vi "AWG Write Multiple PreciseRamps From File.vi"(6 "SourceFolder Path":string, 8 "error in (no error)":errorcluster, 9 "AmpGain":i32=1, 10 "Channel Configurations":T2(array[cluster])=[{"PinNames"=["UP"], "WaveFormFile Name"=""}, {"PinNames"=["DOWN"], "WaveFormFile Name"=""}], 11 "Semiconductor Module Context":T1) -> (0 "error out":errorcluster)   [LabVIEW 2013]
uses:
  <vilib>/NI_TestStand_SemiconductorModule/NI_TestStand_Semiconductor_Module.lvlibp/PinMap/General/SemiconductorModuleContext.ctl
  <instrlib>/niFgen/niFgen.llb/niFgen Write Named Waveform (I16).vi
  <vilib>/NI_TestStand_SemiconductorModule/NI_TestStand_Semiconductor_Module.lvlibp
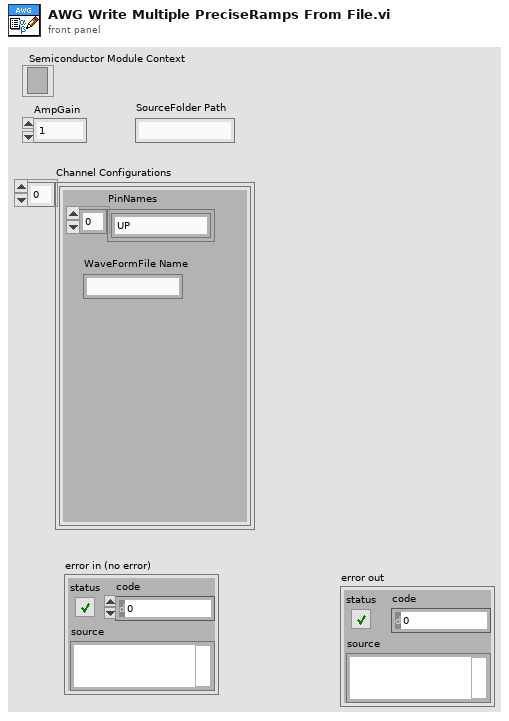
[diagram p1: front panel]
types:
  T1 = typedef "NI_TestStand_Semiconductor_Module.lvlibp/SemiconductorModuleContext.ctl" = refnum<k7>
  T2 = cluster{"PinNames":string[], "WaveFormFile Name":string}[]
  T3 = typedef "PreciseRampWaveformWithName.ctl" = cluster{"Name":string, "Waveform":T4}
  T4 = typedef "PreciseRampWaveform.ctl" = cluster{"Start":dbl, "End":dbl, "Time":dbl}
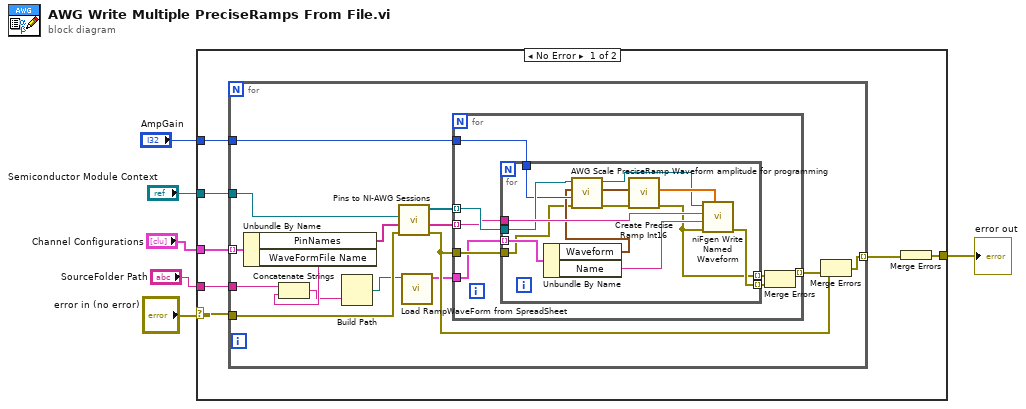
[diagram p0: block diagram]
diagram:
  n1 = case shown="No Error" "error in (no error)" {
    selector: "error in (no error)" -> [w9 w50]
    tunnel: "Channel Configurations" -> [w13 _]
    tunnel: "Semiconductor Module Context" -> [w12 _]
    tunnel: [w10 w50] -> w4
    tunnel: "AmpGain" -> [w8 _]
    tunnel: "SourceFolder Path" -> [w7 _]
    frame No Error {
      n2 = for {
        tunnel: [w23] -> w11 mode=indexing
        tunnel: w13 -> [w26] mode=indexing
        tunnel: w9 -> [w25]
        tunnel: w12 -> [w24]
        tunnel: w8 -> [w20]
        tunnel: w7 -> [w17]
        n3 = Unbundle By Name(w26) -> ("PinNames"=w22:string[], "WaveFormFile Name"=w16:string)
        n4 = Concatenate Strings(w17, w16) -> (w14:string)
        n5 = Build Path(name or relative path=w14) -> (appended path=w15:path)  [unwired: 1 in]
        n6 = call "Pins to NI-AWG Sessions.vi"("error in (no error)"=w25, "Pins"=w22, "Semiconductor Module Context"=w24) -> ("error out"=w21:errorcluster, "Channel Lists"=w27:string[], "Instrument Sessions"=w28:refnum<k15>[])  [unwired: 5 in, 1 out]
        n7 = call "Load RampWaveForm from SpreadSheet.vi"("Path"=w15) -> ("RampWaveForms Array"=w18:T3[])  [unwired: 10 in]
        n8 = for {
          tunnel: w21 -> [w36]
          tunnel: w18 -> [w35]
          tunnel: w28 -> [w32] mode=indexing
          tunnel: w27 -> [w31] mode=indexing
          tunnel: w20 -> [w34]
          tunnel: [w33] -> w19 mode=indexing
          n9 = for {
            tunnel: w36 -> [w41]
            tunnel: w35 -> [w46] mode=indexing
            tunnel: w34 -> [w43]
            tunnel: w32 -> [w44]
            tunnel: w31 -> [w48]
            tunnel: [w47] -> w30 mode=indexing
            tunnel: [w37] -> w29 mode=indexing
            n10 = Unbundle By Name(w46) -> ("Waveform"=w42:T4, "Name"=w39:string)
            n11 = call "AWG Scale PreciseRamp Waveform amplitude for programming.vi"("error in (no error)"=w41, "AmpGain"=w43, "Waveform In"=w42, "Instrument Handle In"=w44) -> ("error out"=w38:errorcluster, "Waveform Out"=w45:T4, "Instrument Handle Out"=w40:refnum<k15>)  [unwired: 5 in]
            n12 = call "Create Precise Ramp Int16.vi"("error in (no error)"=w38, "Waveform"=w45) -> ("error out"=w37:errorcluster, "Waveform Data"=w49:dbl[])  [unwired: 8 in]
            n13 = call-poly <instrlib>:"niFgen Write Named Waveform.vi"("Waveform Data"=w49, "error in (no error)"=w37, "Waveform Name"=w39, "Channel Name"=w48, "Instrument Handle"=w40) -> ("error out"=w47:errorcluster)  [unwired: 4 in, 2 out]
          }
          n14 = Merge Errors(w29, w30) -> (w33:errorcluster)
        }
        n15 = Merge Errors(w21, w19) -> (w23:errorcluster)
      }
      n16 = Merge Errors(w11) -> (w10:errorcluster)
    }
    frame Error {
    }
  }
  "error out" <- w4
